vi "T to V Conversion.vi"(9 "Thermocouple Type":T1 items=["J", "K", "T", "E", "N", "B", "R", "S", "Raw Voltage"], 10 "Temperature Units":T2 items=["Celcius", "Fahrenheit", "Kelvin", "Rankine", "Volts"], 11 "Temperature":dbl) -> (3 "Voltage Out":dbl)   [LabVIEW 2011, in "Simulated Thermocouple Custom Device.lvlib"]
uses:
  Simulated Thermocouple Custom Device.lvlib
  TC Unit Selector.ctl
  TC Selector.ctl
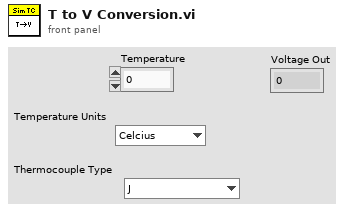
[diagram p1: front panel]
types:
  T1 = typedef "Simulated Thermocouple Custom Device.lvlib/TC Selector.ctl" = u16
  T2 = typedef "Simulated Thermocouple Custom Device.lvlib/TC Unit Selector.ctl" = u16
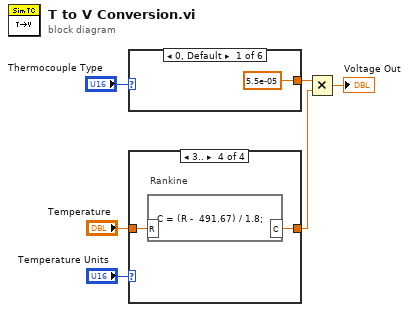
[diagram p0: block diagram]
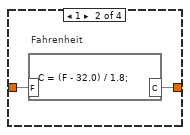
[diagram p3: hidden frame]
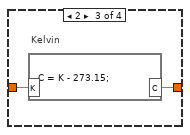
[diagram p4: hidden frame]
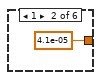
[diagram p5: hidden frame]
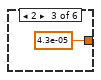
[diagram p6: hidden frame]
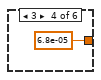
[diagram p7: hidden frame]
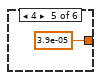
[diagram p8: hidden frame]
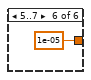
[diagram p9: hidden frame]
diagram:
  n1 = case shown="0, Default" "Thermocouple Type" {
    tunnel: [5.5e-05 ("V") 4.1e-05 ("V") 4.3e-05 ("V") 6.8e-05 ("V") 3.9e-05 ("V") 1e-05 ("V")] -> w3
    frame 0, Default {
    }
    frame 1 {
    }
    frame 2 {
    }
    frame 3 {
    }
    frame 4 {
    }
    frame 5..7 {
    }
  }
  n2 = case shown="3.." "Temperature Units" {
    tunnel: "Temperature" -> [w13 w15 w17 w19]
    tunnel: [w13 w14 w16 w18] -> w1
    frame ..0 {
      # "Celsius"
    }
    frame 1 {
      # "Fahrenheit"
      n3 = formula code="C = (F - 32.0) / 1.8;"("F"=w15) -> ("C"=w14:dbl)
    }
    frame 2 {
      # "Kelvin"
      n4 = formula code="C = K - 273.15;"("K"=w17) -> ("C"=w16:dbl)
    }
    frame 3.. {
      # "Rankine"
      n5 = formula code="C = (R -  491.67) / 1.8;"("R"=w19) -> ("C"=w18:dbl)
    }
  }
  n6 = Multiply(x=w3, y=w1) -> (x*y=→"Voltage Out":dbl)
